vi "Main_Console.vi"(0 "Log_File_Folder":path caption="Log File Folder", 5 "Value_In":dbl caption="Value In" min=-4294967295.0 max=4294967296.0, 7 "Command":T1(ring), 9 "Stop":bool) -> (4 "Value_Out":string caption="Value Out")   [LabVIEW 2023]
doc: "This VI is the Console VI which communicate with Sour_Meas_instrument."
uses:
  <vilib>/Utility/file.llb/Write Delimited Spreadsheet (string).vi
panel:
  out "Error_Out":errorcluster
  in  "Error_In":errorcluster
  # "Control"
  # "Display"
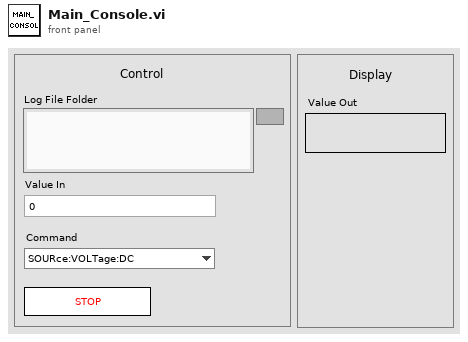
[diagram p1: front panel]
types:
  T1 = enum16{"SOURce:VOLTage:DC", "SOURce:CURRent:DC", "MEASure:VOLTage:DC?", "MEASure:CURRent:DC?"}
  T2 = enum16{"Left Button", "Center Button", "Right Button", "Window Close"}
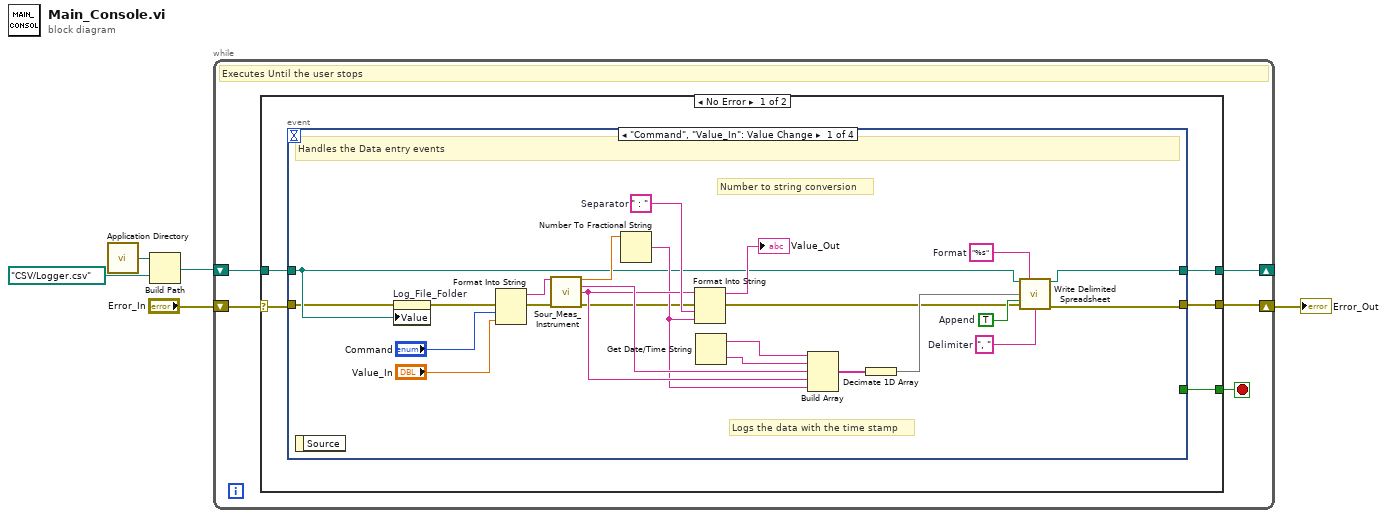
[diagram p0: block diagram]
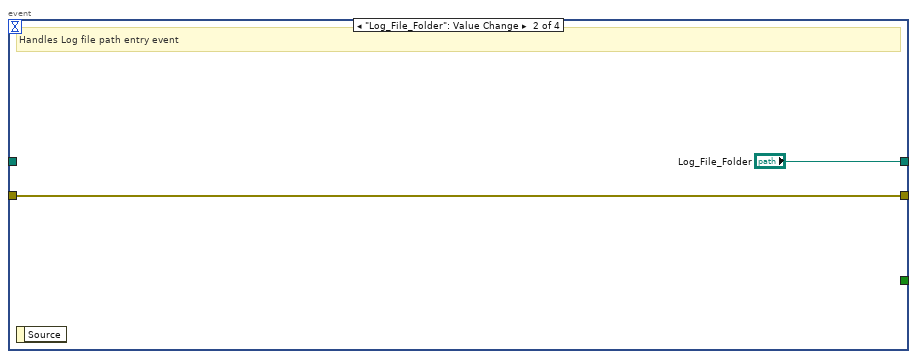
[diagram p2: hidden frame]
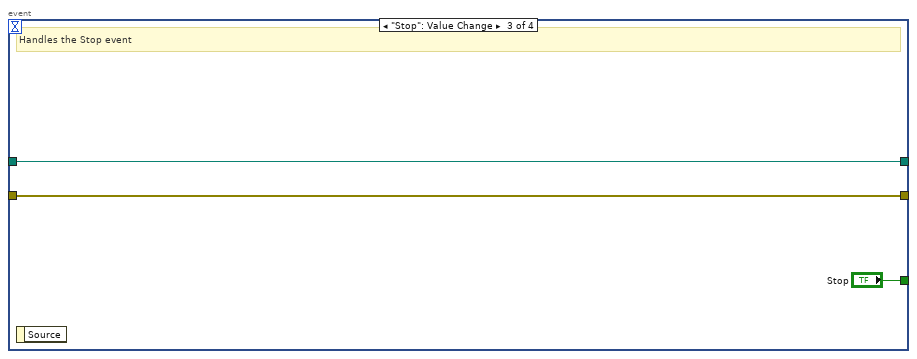
[diagram p3: hidden frame]
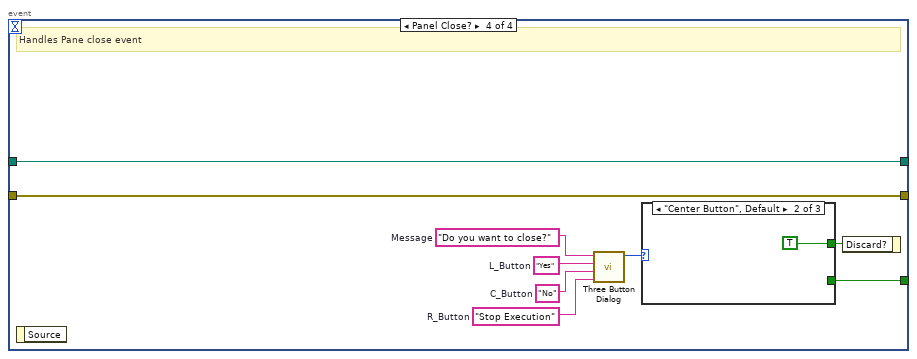
[diagram p4: hidden frame]
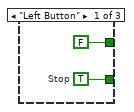
[diagram p5: hidden frame]
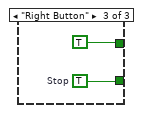
[diagram p6: hidden frame]
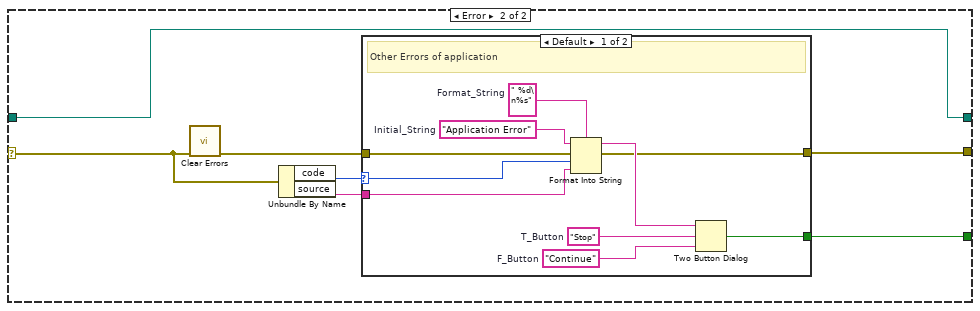
[diagram p7: hidden frame]
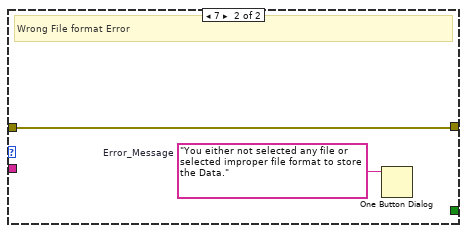
[diagram p8: hidden frame]
diagram:
  n1 = call <vilib>:"Application Directory.vi"() -> ("Application Directory"=w2:path)
  n2 = Build Path(base path=w2, name or relative path=path "CSV/Logger.csv") -> (appended path=w3:path)
  n3 = while {
    shift-right: [w8] -> w5
    shift-left: "Error_In" -> [w9]
    shift-right: [w7] -> _
    shift-left: w3 -> [w6]
    stop <- w10 stop-if-true
    # "Executes Until the user stops"
    n4 = case shown="No Error" w9 {
      selector: w9 -> [w14 w65]
      tunnel: [w15 w62] -> w10
      tunnel: [w13 w60] -> w8
      tunnel: [w12 w59] -> w7
      tunnel: w6 -> [w11 w59]
      frame No Error {
        n5 = event shown="[0] \"Command\", \"Value_In\": Value Change" {
          selector: _ -> [_ _ _ _]
          dyn-events: _ -> [_ _ _ _]
          timeout: _ -> [_ _ _ _]
          tunnel: [_ _ "Stop" w47] -> w15
          tunnel: w14 -> [w17 w40 w43 w46]
          tunnel: [w21 w40 w43 w46] -> w13
          tunnel: [w22 "Log_File_Folder" w44 w45] -> w12
          tunnel: w11 -> [w18 _ w44 w45]
          event "Command", "Value_In": Value Change {
            w31 = TRUE  # Append
            w37 = "%s"  # Format
            w28 = ", "  # Delimiter
            w38 = " : "  # Separator
            # "Number to string conversion"
            # "Logs the data with the time stamp"
            # "Handles the Data entry events"
            n6 = event-data() -> ()  [unwired: 1 in, 1 out]
            n7 = property on="Log_File_Folder" class="Path"(error in=w17, "Value"=w18) -> (error out=w16:errorcluster)  [unwired: 1 in, 1 out]
            n8 = Format Into String(error in=w16, "Command", "Value_In") -> (resulting string=w24:string, error out=w23:errorcluster)  [unwired: 2 in]
            n9 = call "Sour_Meas_Instrument.vi"("Command"=w24, "Error_In"=w23) -> ("Responce"=w39:dbl, "Action"=w36:string, "Parameter"=w35:string, "Error_Out"=w26:errorcluster)  [unwired: 10 in]
            n10 = Number To Fractional String(number=w39) -> (F-format string=w34:string)  [unwired: 3 in]
            n11 = Format Into String(initial string=w35, error in=w26, w38, w34) -> (resulting string=→"Value_Out":string, error out=w20:errorcluster)  [unwired: 1 in]
            n12 = Get Date/Time String() -> (date string=w30:string, time string=w29:string)  [unwired: 3 in]
            n13 = Build Array(w30, w29, w36, w35, w34) -> (w33:string[])
            n14 = Decimate 1D Array(w33) -> (w32:string[])
            n15 = call-poly <vilib>:"Write Delimited Spreadsheet.vi"("file path (dialog if empty)"=w18, "format (%s)"=w37, "1D data"=w32, "append to file? (new file:F)"=w31, "error in (no error)"=w20, "delimiter (\\t)"=w28) -> ("new file path (Not A Path if cancelled)"=w22:path, "error out"=w21:errorcluster)  [unwired: 8 in]
          }
          event "Log_File_Folder": Value Change {
            # "Handles Log file path entry event"
            n16 = event-data() -> ()  [unwired: 1 in, 1 out]
          }
          event "Stop": Value Change {
            # "Handles the Stop event"
            n17 = event-data() -> ()  [unwired: 1 in, 1 out]
          }
          event Panel Close? {
            w50 = "Stop Execution"  # R_Button
            w51 = "No"  # C_Button
            w52 = "Yes"  # L_Button
            w53 = "Do you want to close?"  # Message
            # "Handles Pane close event"
            n18 = event-data() -> ()  [unwired: 1 in, 1 out]
            n19 = call <vilib>:"Three Button Dialog.vi"("Right Button Text (\"Cancel\")"=w50, "Center Button Text (\"No\")"=w51, "Left Button Text (\"Yes\")"=w52, "message"=w53) -> ("Which Button?"=w49:T2)  [unwired: 7 in]
            n20 = case shown="\"Center Button\", Default" w49 {
              tunnel: [FALSE TRUE TRUE] -> w48
              tunnel: [w54 _ w58] -> w47
              frame "Left Button" {
                w54 = TRUE  # Stop
              }
              frame "Center Button", Default {
              }
              frame "Right Button" {
                w58 = TRUE  # Stop
              }
            }
            n21 = event-data ("Event Filter Node")("Discard?"=w48) -> ()  [unwired: 1 in, 1 out]
          }
        }
      }
      frame Error {
        n22 = call <vilib>:"Clear Errors.vi"("error in (no error)"=w65) -> ("error out"=w61:errorcluster)  [unwired: 5 in, 1 out]
        n23 = Unbundle By Name(w65) -> ("code"=w64:i32, "source"=w63:string)
        n24 = case shown="Default" w64 {
          selector: w64 -> [w75 _]
          tunnel: w63 -> [w66 _]
          tunnel: [w71 _] -> w62
          tunnel: w61 -> [w69 w76]
          tunnel: [w68 w76] -> w60
          frame Default {
            w67 = " %d\n%s"  # Format_String
            w70 = "Application Error"  # Initial_String
            w72 = "Stop"  # T_Button
            w73 = "Continue"  # F_Button
            # "Other Errors of application"
            n25 = Format Into String(format string=w67, initial string=w70, error in=w69, w75, w66) -> (resulting string=w74:string, error out=w68:errorcluster)
            n26 = Two Button Dialog(message=w74, 1:w73, 2:w72) -> (T button?=w71:bool)
          }
          frame 7 {
            w77 = "You either not selected any file or selected improper file format to store the Data."  # Error_Message
            # "Wrong File format Error"
            n27 = One Button Dialog(message=w77) -> ()  [unwired: 1 in, 1 out]
          }
        }
      }
    }
  }
  "Error_Out" <- w5
